vi "Move motors.vi"(8 "Error In":errorcluster, 9 "Boolean_Array":bool[](array[boolean]), 10 "Numeric_Array":dbl[](array[numeric]), 11 "VISA resource name":refnum<visa-resource-name>) -> (0 "Error Out":errorcluster)   [LabVIEW 2017]
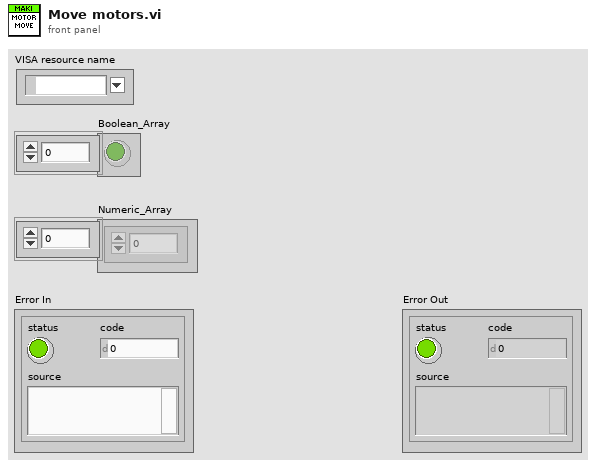
[diagram p1: front panel]
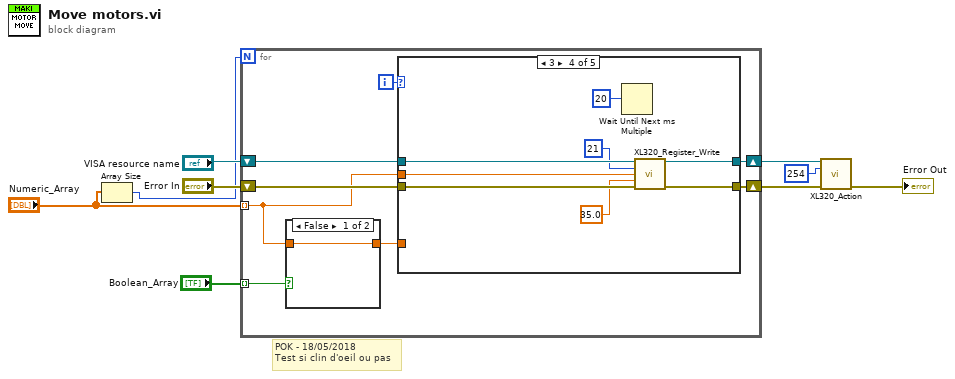
[diagram p0: block diagram]
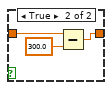
[diagram p2: hidden frame]
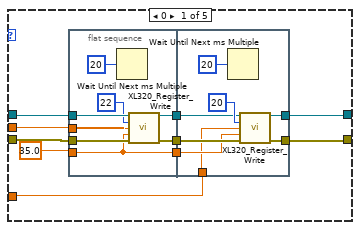
[diagram p3: hidden frame]
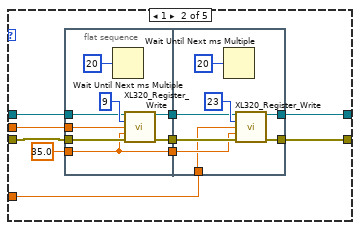
[diagram p4: hidden frame]
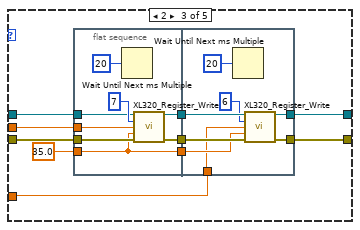
[diagram p5: hidden frame]
diagram:
  # "POK - 18/05/2018\nTest si clin d'oeil ou pas"
  n1 = Array Size(array="Numeric_Array") -> (size(s)=w7:i32)
  n2 = for {
    N: w7 -> [_]
    shift-right: [w17] -> w4
    shift-left: "Error In" -> [w16]
    shift-right: [w14] -> w1
    shift-left: "VISA resource name" -> [w15]
    tunnel: "Numeric_Array" -> [w10] mode=indexing
    tunnel: "Boolean_Array" -> [w12] mode=indexing
    i -> [w13]
    n3 = case shown="False" w12 {
      tunnel: w10 -> [w18 w21]
      tunnel: [w18 w19] -> w11
      frame False {
      }
      frame True {
        n4 = Subtract(x=w21, y=300.0) -> (x-y=w19:dbl)
      }
    }
    n5 = case shown="3" w13 {
      tunnel: [w27 w48 w79 w104 w109] -> w17
      tunnel: w16 -> [w26 w54 w78 w106 w109]
      tunnel: w15 -> [w25 w55 w77 w107 w108]
      tunnel: [w28 w49 w80 w103 w108] -> w14
      tunnel: w11 -> [w22 w50 w75 _ _]
      tunnel: w10 -> [w23 w51 w74 w105 _]
      frame 0 {
        n6 = flat-sequence {
          tunnel: w25 -> [w39]
          tunnel: w26 -> [w38]
          tunnel: [w37] -> w31
          tunnel: [w36] -> w30
          tunnel: 35.0 -> [w34]
          tunnel: [w34] -> w29
          tunnel: w23 -> [w33]
          tunnel: w31 -> [w46]
          tunnel: w30 -> [w45]
          tunnel: [w43] -> w28
          tunnel: [w42] -> w27
          tunnel: w29 -> [w41]
          tunnel: w22 -> [w40]
          frame #0 {
            n7 = Wait Until Next ms Multiple(millisecond multiple=u32 20 ("n millisecondes")) -> ()  [unwired: 1 out]
            n8 = call <instrlib>:"XL320_Register_Write.vi"("VISA resource name"=w39, "Motor ID (0)"=u8 22, "Goal Position (150 deg)"=w33, "Goal Speed (RPM)"=w34, "error in (no error)"=w38) -> ("VISA resource name out"=w37:refnum<visa-resource-name>, "error out"=w36:errorcluster)  [unwired: 8 in, 1 out]
          }
          frame #1 {
            n9 = Wait Until Next ms Multiple(millisecond multiple=u32 20 ("n millisecondes")) -> ()  [unwired: 1 out]
            n10 = call <instrlib>:"XL320_Register_Write.vi"("VISA resource name"=w46, "Motor ID (0)"=u8 20, "Goal Position (150 deg)"=w40, "Goal Speed (RPM)"=w41, "error in (no error)"=w45) -> ("VISA resource name out"=w43:refnum<visa-resource-name>, "error out"=w42:errorcluster)  [unwired: 8 in, 1 out]
          }
        }
      }
      frame 1 {
        n11 = flat-sequence {
          tunnel: w55 -> [w64]
          tunnel: w54 -> [w63]
          tunnel: [w62] -> w57
          tunnel: [w61] -> w56
          tunnel: 35.0 -> [w59]
          tunnel: [w59] -> w52
          tunnel: w51 -> [w58]
          tunnel: w57 -> [w72]
          tunnel: w56 -> [w71]
          tunnel: [w69] -> w49
          tunnel: [w68] -> w48
          tunnel: w52 -> [w67]
          tunnel: w50 -> [w66]
          frame #0 {
            n12 = Wait Until Next ms Multiple(millisecond multiple=u32 20 ("n millisecondes")) -> ()  [unwired: 1 out]
            n13 = call <instrlib>:"XL320_Register_Write.vi"("VISA resource name"=w64, "Motor ID (0)"=u8 9, "Goal Position (150 deg)"=w58, "Goal Speed (RPM)"=w59, "error in (no error)"=w63) -> ("VISA resource name out"=w62:refnum<visa-resource-name>, "error out"=w61:errorcluster)  [unwired: 8 in, 1 out]
          }
          frame #1 {
            n14 = Wait Until Next ms Multiple(millisecond multiple=u32 20 ("n millisecondes")) -> ()  [unwired: 1 out]
            n15 = call <instrlib>:"XL320_Register_Write.vi"("VISA resource name"=w72, "Motor ID (0)"=u8 23, "Goal Position (150 deg)"=w66, "Goal Speed (RPM)"=w67, "error in (no error)"=w71) -> ("VISA resource name out"=w69:refnum<visa-resource-name>, "error out"=w68:errorcluster)  [unwired: 8 in, 1 out]
          }
        }
      }
      frame 2 {
        n16 = flat-sequence {
          tunnel: w77 -> [w90]
          tunnel: w78 -> [w89]
          tunnel: [w88] -> w83
          tunnel: [w87] -> w82
          tunnel: 35.0 -> [w85]
          tunnel: [w85] -> w81
          tunnel: w74 -> [w84]
          tunnel: w83 -> [w99]
          tunnel: w82 -> [w98]
          tunnel: [w97] -> w80
          tunnel: [w96] -> w79
          tunnel: w81 -> [w95]
          tunnel: w75 -> [w94]
          frame #0 {
            n17 = Wait Until Next ms Multiple(millisecond multiple=u32 20 ("n millisecondes")) -> ()  [unwired: 1 out]
            n18 = call <instrlib>:"XL320_Register_Write.vi"("VISA resource name"=w90, "Motor ID (0)"=u8 7, "Goal Position (150 deg)"=w84, "Goal Speed (RPM)"=w85, "error in (no error)"=w89) -> ("VISA resource name out"=w88:refnum<visa-resource-name>, "error out"=w87:errorcluster)  [unwired: 8 in, 1 out]
          }
          frame #1 {
            n19 = Wait Until Next ms Multiple(millisecond multiple=u32 20 ("n millisecondes")) -> ()  [unwired: 1 out]
            n20 = call <instrlib>:"XL320_Register_Write.vi"("VISA resource name"=w99, "Motor ID (0)"=u8 6, "Goal Position (150 deg)"=w94, "Goal Speed (RPM)"=w95, "error in (no error)"=w98) -> ("VISA resource name out"=w97:refnum<visa-resource-name>, "error out"=w96:errorcluster)  [unwired: 8 in, 1 out]
          }
        }
      }
      frame 3 {
        n21 = Wait Until Next ms Multiple(millisecond multiple=u32 20 ("n millisecondes")) -> ()  [unwired: 1 out]
        n22 = call <instrlib>:"XL320_Register_Write.vi"("VISA resource name"=w107, "Motor ID (0)"=u8 21, "Goal Position (150 deg)"=w105, "Goal Speed (RPM)"=35.0, "error in (no error)"=w106) -> ("VISA resource name out"=w103:refnum<visa-resource-name>, "error out"=w104:errorcluster)  [unwired: 8 in, 1 out]
      }
      frame Default {
      }
    }
  }
  n23 = call <instrlib>:"XL320_Action.vi"("VISA resource name"=w1, "Motor ID (0)"=u8 254, "error in (no error)"=w4) -> ("error out"=→"Error Out":errorcluster)  [unwired: 10 in, 2 out]
